vi "Laurel Modbus Initialize.vi"(8 "error in (no error)":errorcluster, 11 "Remote IP Address":string) -> (0 "error out":errorcluster, 3 "Modbus Master out":refnum<class "Modbus Master.lvclass">)   [LabVIEW 2020]
uses:
  <vilib>/NI/Modbus Library/API/Master/Modbus Master.lvclass
  <vilib>/NI/Modbus Library/API/Wrapper/Create TCP Master.vi
  <vilib>/NI/Modbus Library/API/Wrapper/API Main.lvlib
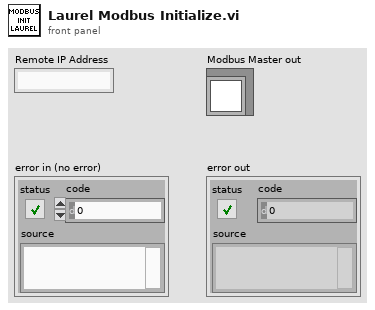
[diagram p1: front panel]
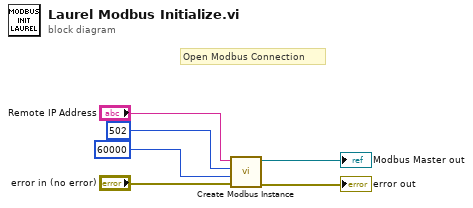
[diagram p0: block diagram]
diagram:
  # "Open Modbus Connection"
  n1 = call-poly <vilib>:"Create Modbus Instance.vi"("error in"="error in (no error)", "connect timeout ms"=60000, "port (502)"=u16 502, "address"="Remote IP Address") -> ("error out"=→"error out":errorcluster, "TCP master instance"=→"Modbus Master out":refnum<class "Modbus Master.lvclass">)  [unwired: 6 in]
